vi "solar_probe.vi"(11 "solar":refnum<class "solar.lvclass">) -> (2 "Value String":string, 3 "Boolean":bool)   [LabVIEW 2018, in "solar.lvclass"]
doc: "This is the default solar.lvclass probe."
uses:
  solar.lvclass
  solar_ctl SOLAR Global.ctl
  solar_ctl Target Global.ctl
  voyager/solar_voy_ctl Voyager Refnum.ctl
  qtimer/solar_qtimer_ctl Refnum.ctl
panel:
  in  "Tab Control":enum32{"LVClass", "App Info"}(tab)
  out "Targets":string[][](table)
  out "App Info":string[][](table)
  out "SOLAR":T1
  out "LVClass":string
  out "Name":string
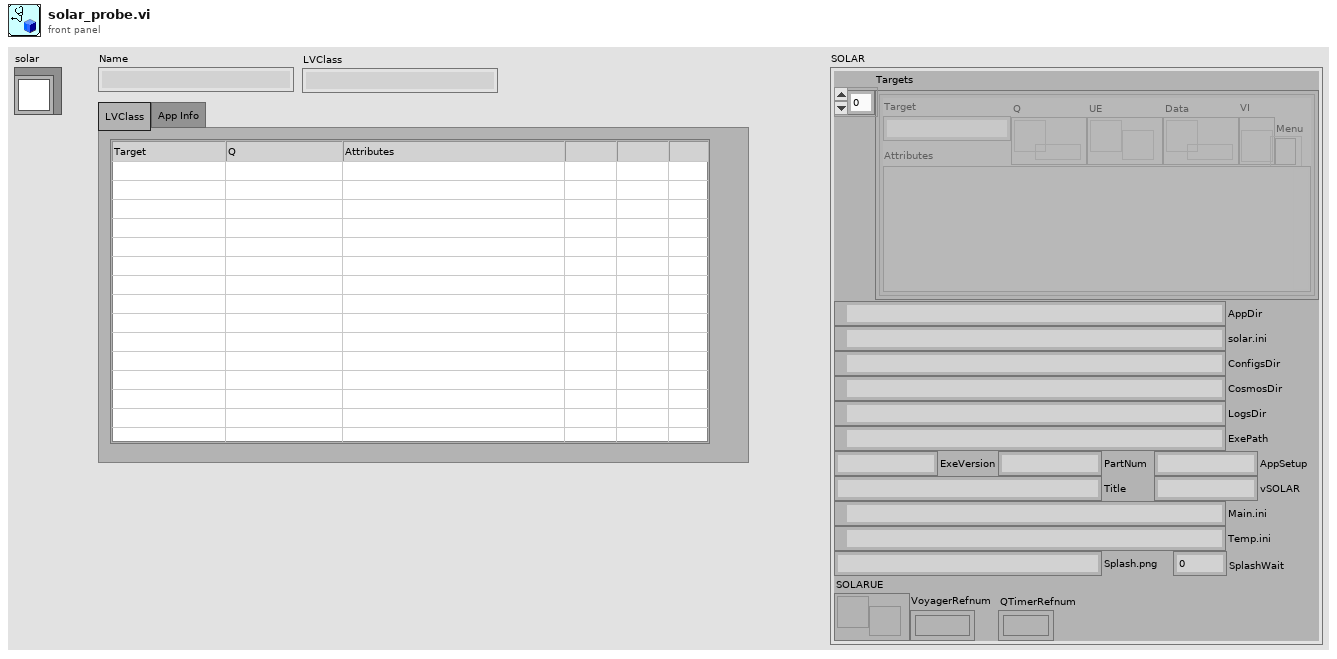
[diagram p1: front panel]
types:
  T1 = typedef "solar_ctl SOLAR Global.ctl" = cluster{"Targets":T2[], "AppDir":path, "solar.ini":path, "ConfigsDir":path, "CosmosDir":path, "LogsDir":path, "ExePath":path, "ExeVersion":string, "PartNum":string, "AppSetup":string, "Title":string, "Main.ini":path, "Temp.ini":path, "vSOLAR":string, "Splash.png":string, "SplashWait":i32, "SOLARUE":refnum<user-event>, "VoyagerRefnum":T3, "QTimerRefnum":T4}
  T2 = typedef "solar_ctl Target Global.ctl" = cluster{"Target":string, "Q":refnum<queue>, "UE":refnum<user-event>, "VI":refnum<vi>, "Menu":refnum<k9>, "Data":refnum<data-value>, "Attributes":variant}
  T3 = typedef "solar_voy_ctl Voyager Refnum.ctl" = refnum<k1>
  T4 = typedef "solar_qtimer_ctl Refnum.ctl" = refnum<k1>
  T5 = typedef "solar_ctl SOLAR Refnum.ctl" = refnum<k1>
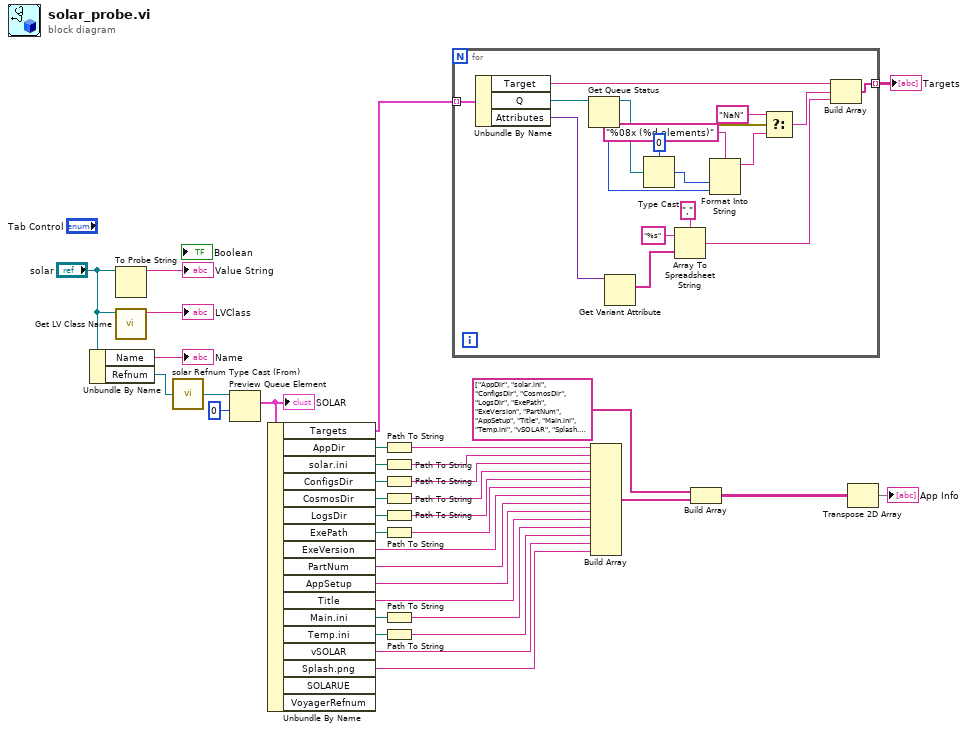
[diagram p0: block diagram]
diagram:
  n1 = Unbundle By Name("solar") -> ("Name"=→"Name":string, "Refnum"=w32:T5)
  n2 = To Probe String(7:"solar") -> (3:→"Value String":string)  [unwired: 2 in, 1 out]
  n3 = call <vilib>:"Get LV Class Name.vi"("object"="solar") -> ("class name"=→"LVClass":string)  [unwired: 9 in, 1 out]
  n4 = call "solar Refnum Type Cast (From).vi"("Refnum"=w32) -> ("SOLAR"=w31:refnum<queue>)
  n5 = Preview Queue Element(queue=w31, timeout in ms (-1)=0) -> (element=w29:T1)  [unwired: 1 in, 3 out]
  "SOLAR" <- w29
  n6 = Unbundle By Name(w29) -> ("Targets"=w1:T2[], "AppDir"=w28:path, "solar.ini"=w27:path, "ConfigsDir"=w26:path, "CosmosDir"=w25:path, "LogsDir"=w24:path, "ExePath"=w23:path, "ExeVersion"=w14:string, "PartNum"=w13:string, "AppSetup"=w12:string, "Title"=w11:string, "Main.ini"=w22:path, "Temp.ini"=w21:path, "vSOLAR"=w8:string, "Splash.png"=w7:string)  [unwired: 2 out]
  n7 = Path To String(path=w28) -> (string=w20:string)
  n8 = Path To String(path=w27) -> (string=w19:string)
  n9 = Path To String(path=w26) -> (string=w18:string)
  n10 = Path To String(path=w25) -> (string=w17:string)
  n11 = Path To String(path=w24) -> (string=w16:string)
  n12 = Path To String(path=w23) -> (string=w15:string)
  n13 = Path To String(path=w22) -> (string=w10:string)
  n14 = Path To String(path=w21) -> (string=w9:string)
  n15 = for {
    tunnel: w1 -> [w54] mode=indexing
    tunnel: [w51] -> w2 mode=indexing
    n16 = Unbundle By Name(w54) -> ("Target"=w52:string, "Q"=w53:refnum<queue>, "Attributes"=w41:variant)
    n17 = Get Queue Status(queue=w53) -> (queue out=w48:refnum<queue>, error out=w49:errorcluster, # elements in queue=w50:i32)  [unwired: 2 in, 5 out]
    n18 = Get Variant Attribute(Variant=w41) -> (names=w40:string[])  [unwired: 3 in, 3 out]
    n19 = Type Cast(type=u32 0 ("# elements in queue"), x=w48) -> (*(type *) &x=w46:u32)
    n20 = Array To Spreadsheet String(delimiter (Tab)=",", array=w40, 3:"%s" ("format string")) -> (spreadsheet string=w37:string)
    n21 = Format Into String(format string="%08x (%d elements)", w46, w50) -> (resulting string=w44:string)  [unwired: 2 in, 1 out]
    n22 = Select(t="NaN", s=w49, f=w44) -> (s? t:f=w42:string)
    n23 = Build Array(w52, w42, w37) -> (w51:string[])
  }
  "Targets" <- w2
  n24 = Build Array(w20, w19, w18, w17, w16, w15, w14, w13, w12, w11, w10, w9, w8, w7) -> (w6:string[])
  n25 = Build Array(string[] ["AppDir", "solar.ini", "ConfigsDir", "CosmosDir", "LogsDir", "ExePath", "ExeVersion", "PartNum", "AppSetup", "Title", "Main.ini", "Temp.ini", "vSOLAR", "Splash.png"], w6) -> (w4:string[][])
  n26 = Transpose 2D Array(2D array=w4) -> (transposed array=→"App Info":string[][])
